vi "TEST_DSP.vi"() -> ()   [LabVIEW 2019]
panel:
  in  "error in (no error) 2":errorcluster
  out "Waveform Chart":cluster{"Data[0]":dbl, "Data[1]":dbl}(graph)
  in  "Voltage":dbl=5.0
  in  "Current":dbl=1.0
  in  "OCP Level":dbl=5.0 format="%#_13g"
  in  "OVP Level":dbl=10.0 format="%#_13g"
  out "Read Data":string="iDRC,DSP1500-30WE,702648,1.03.42\n"
  in  "port":refnum<visa-resource-name>="TCPIP0::192.168.0.14::HISLIP0::INSTR"
  in  "conntect":bool
  in  "disconntect":bool
  in  "READ":bool
  in  "STOP":bool
  in  "ON":bool
  in  "OFF":bool
  out "error out 3":errorcluster
  # "iDRC"
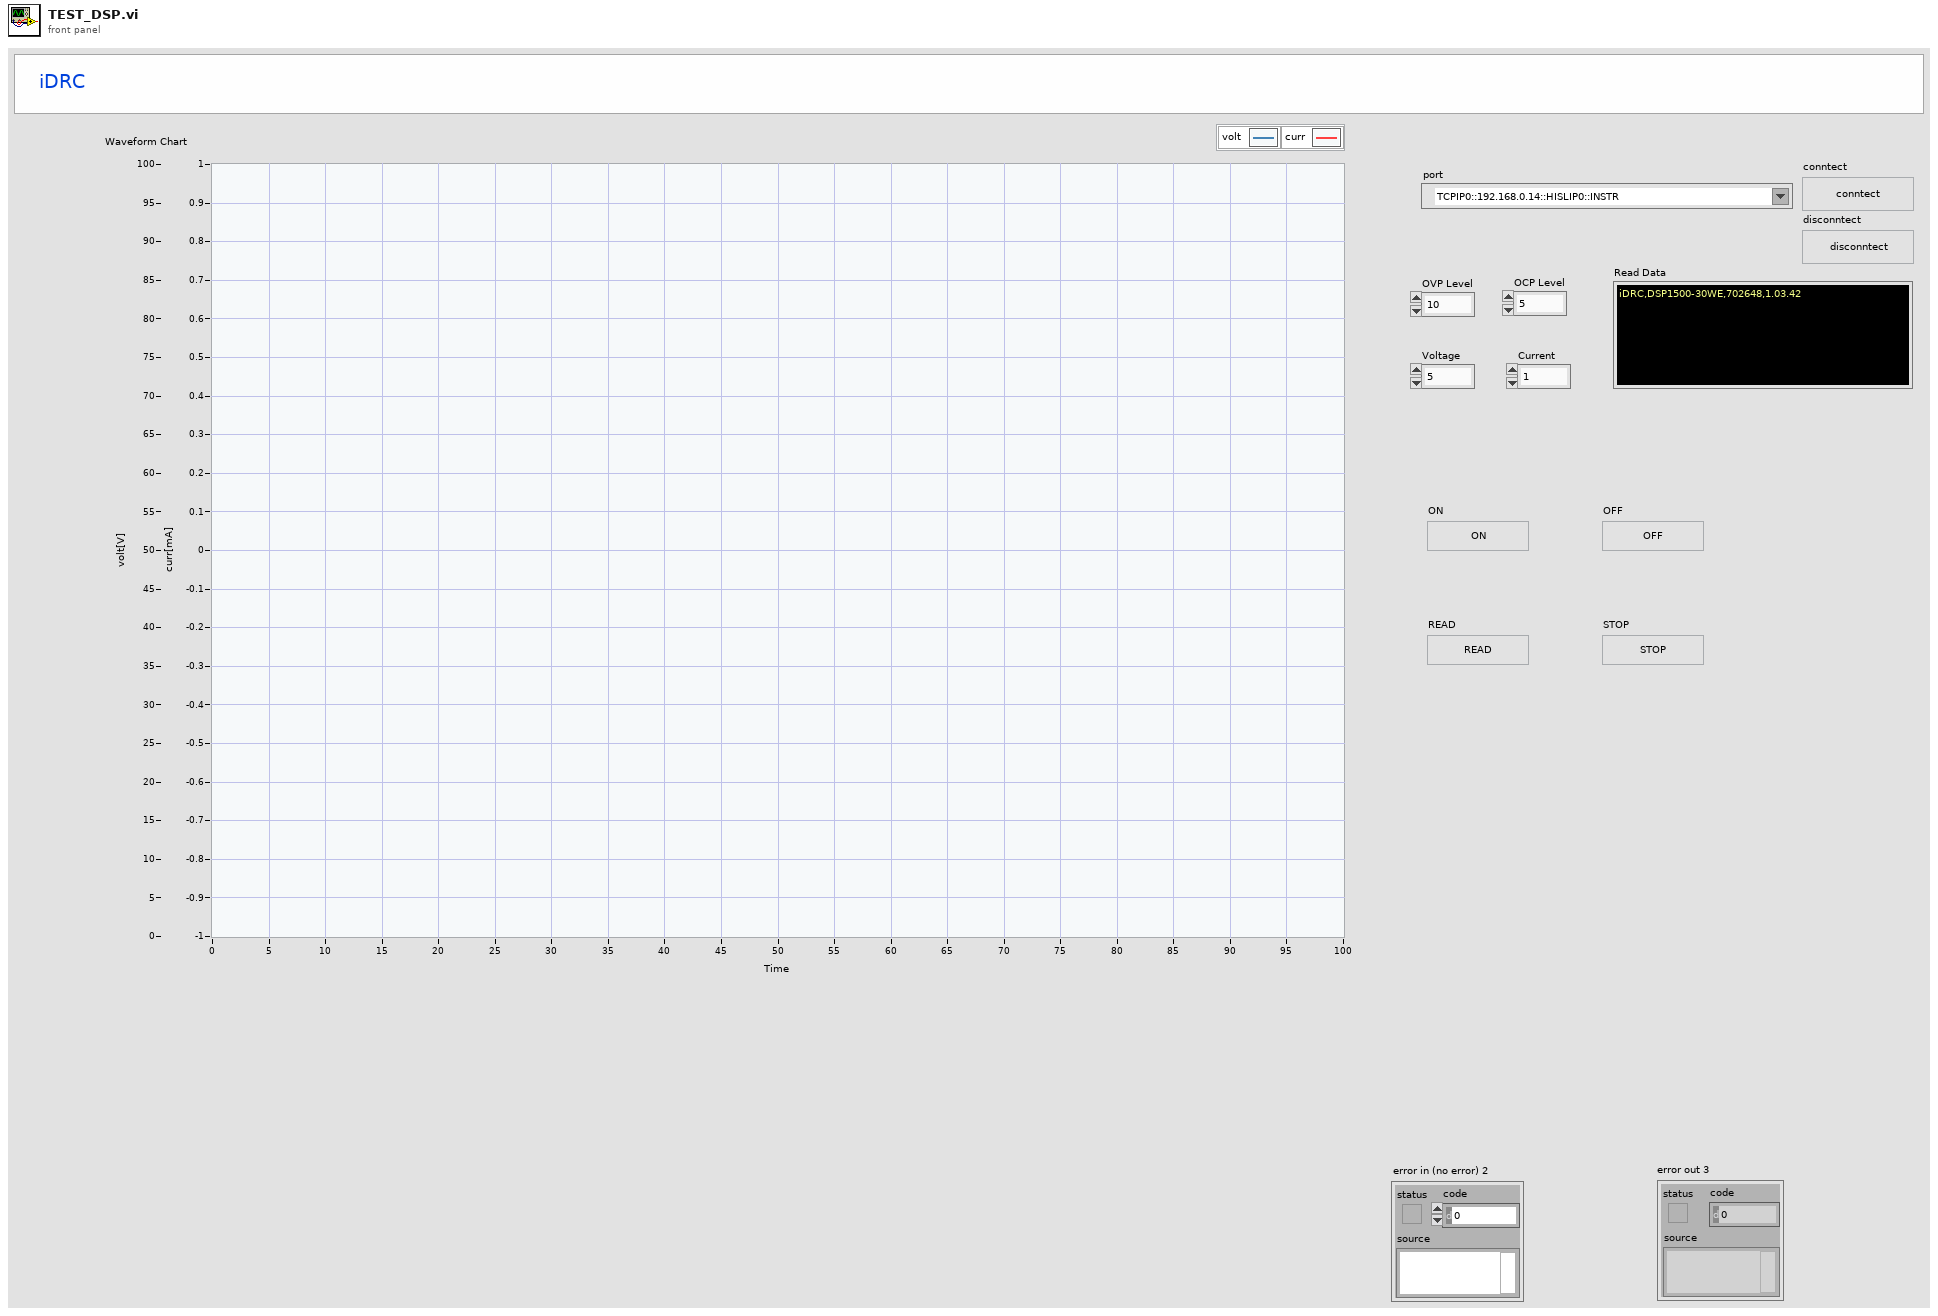
[diagram p1: front panel]
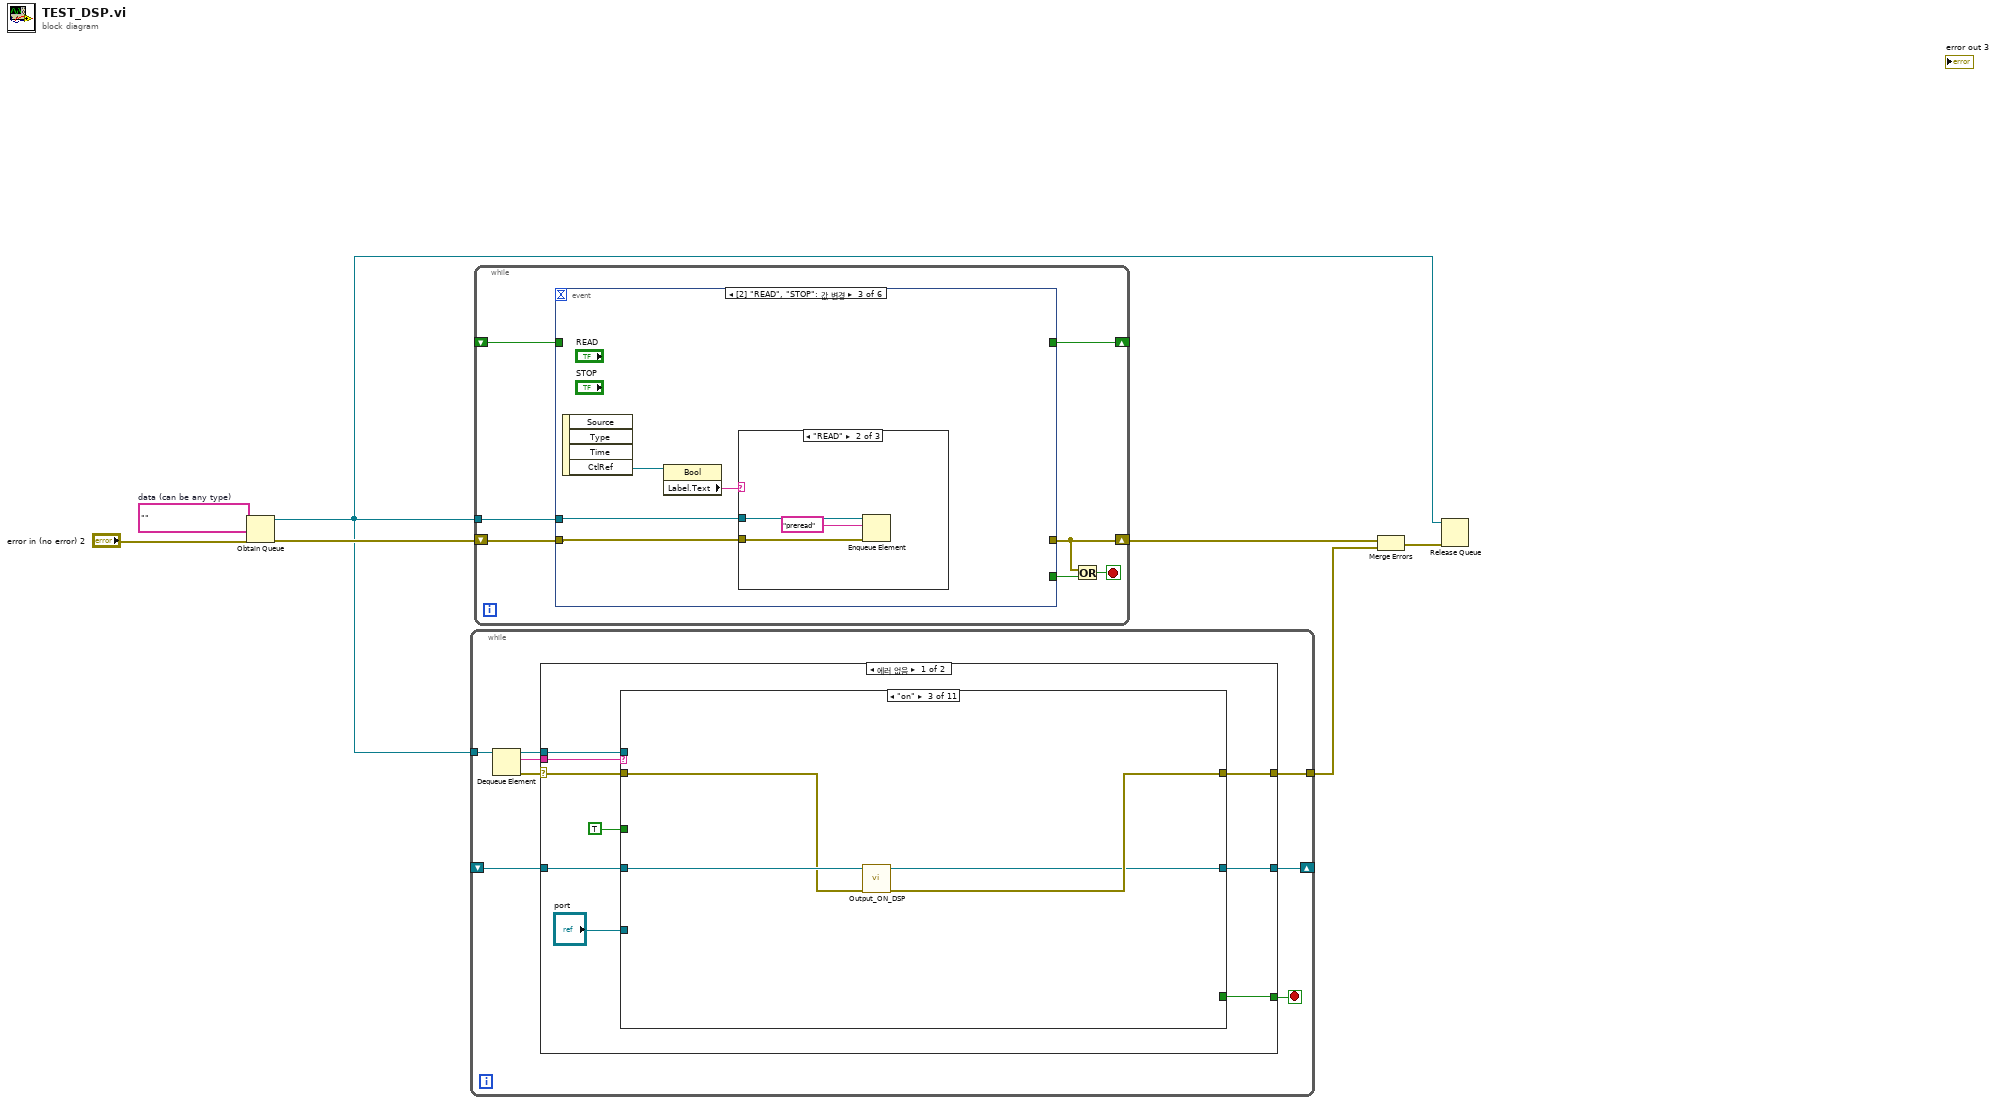
[diagram p0: block diagram]
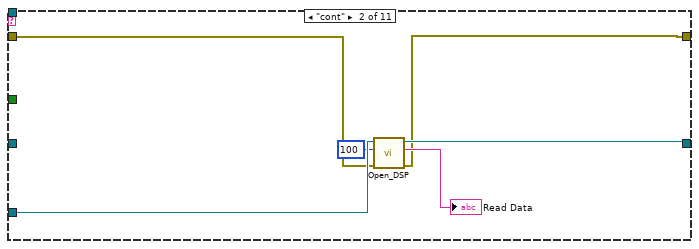
[diagram p3: hidden frame]
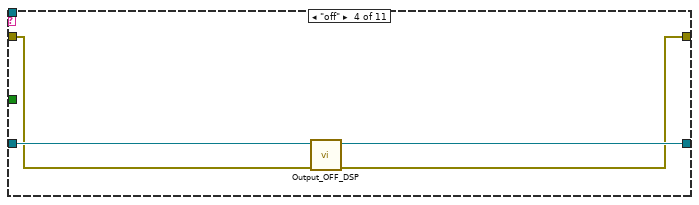
[diagram p4: hidden frame]
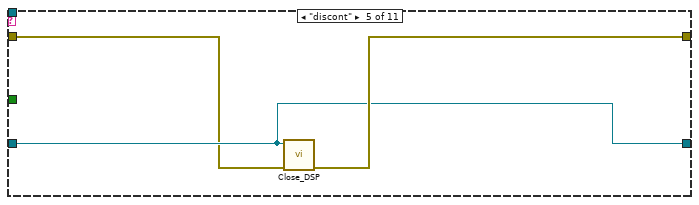
[diagram p5: hidden frame]
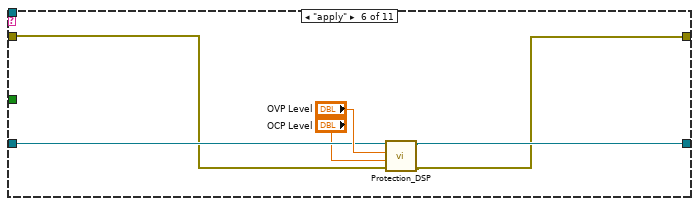
[diagram p6: hidden frame]
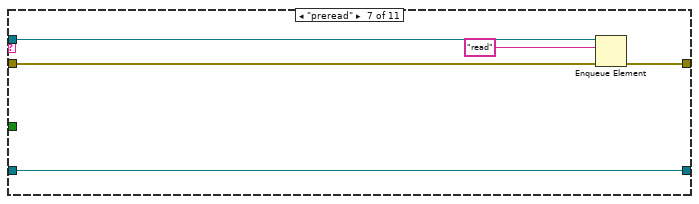
[diagram p7: hidden frame]
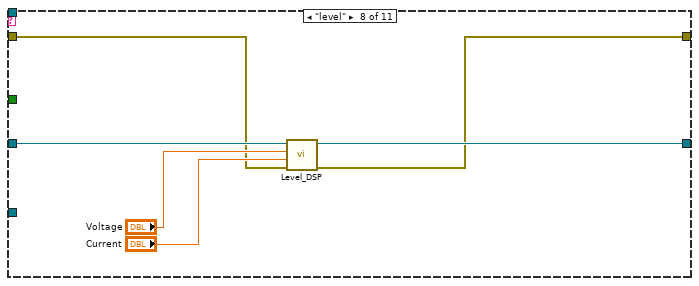
[diagram p8: hidden frame]
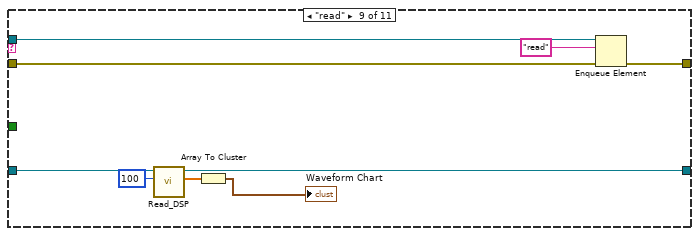
[diagram p9: hidden frame]
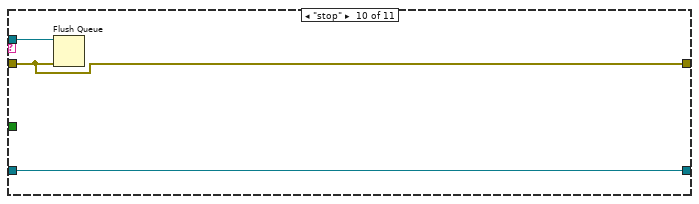
[diagram p10: hidden frame]
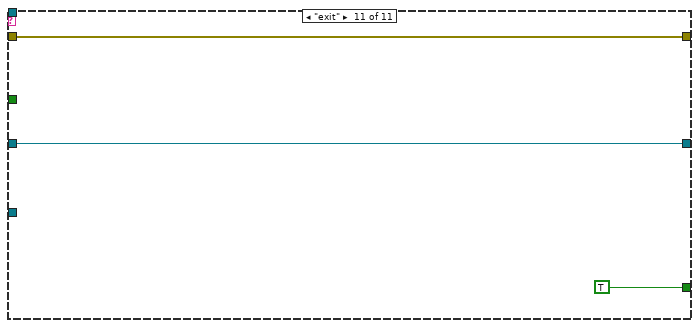
[diagram p11: hidden frame]
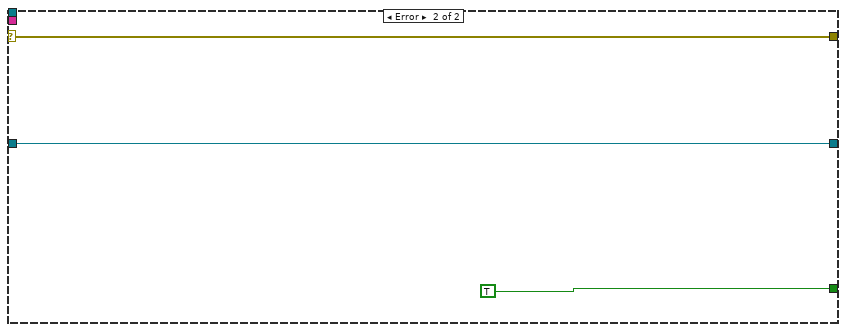
[diagram p12: hidden frame]
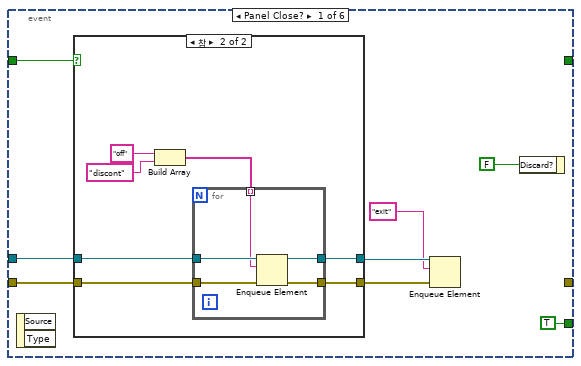
[diagram p13: hidden frame]
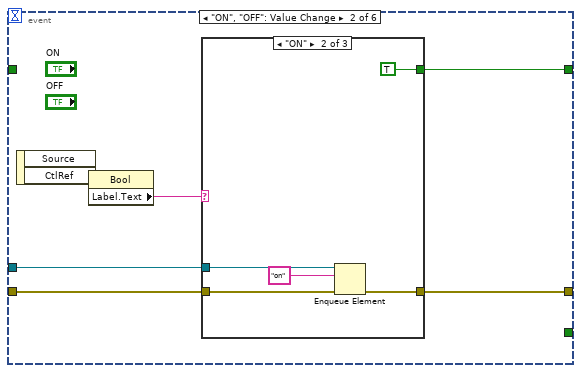
[diagram p15: hidden frame]
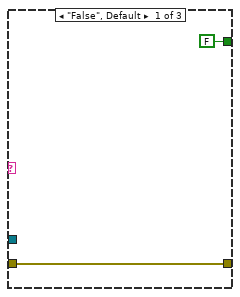
[diagram p16: hidden frame]
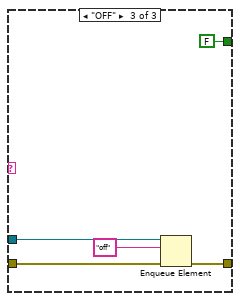
[diagram p17: hidden frame]
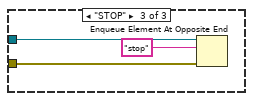
[diagram p19: hidden frame]
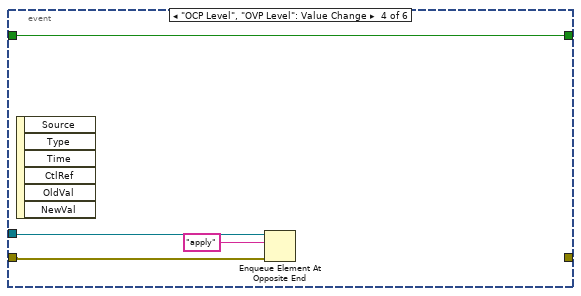
[diagram p20: hidden frame]
diagram:
  w6 = ""  # data (can be any type)
  n1 = Obtain Queue(element data type=w6, error in (no error)="error in (no error) 2") -> (queue out=w5:refnum<queue>, error out=w7:errorcluster)  [unwired: 3 in, 1 out]
  n2 = while {
    tunnel: w5 -> [w15]
    tunnel: [w10] -> w2
    shift-right: [w9] -> _
    shift-left: _ -> [w8]
    stop <- w12 stop-if-true
    n3 = Dequeue Element(queue=w15) -> (queue out=w11:refnum<queue>, element=w13:string, error out=w14:errorcluster)  [unwired: 2 in, 1 out]
    n4 = case shown="에러 없음" w14 {
      selector: w14 -> [w22 w77]
      tunnel: w13 -> [w24 _]
      tunnel: [w21 TRUE] -> w12
      tunnel: w11 -> [w23 _]
      tunnel: [w20 w77] -> w10
      tunnel: [w19 w76] -> w9
      tunnel: w8 -> [w18 w76]
      frame No Error {
        n5 = case shown="\"on\"" w24 {
          tunnel: w23 -> [_ _ _ _ _ _ w53 _ w69 w72 _]
          tunnel: w22 -> [w26 w29 w35 w38 w41 w46 w52 w56 w65 w71 w73]
          tunnel: [_ _ _ _ _ _ _ _ _ _ TRUE] -> w21
          tunnel: [w26 w28 w34 w37 w43 w45 w50 w55 w68 w71 w73] -> w20
          tunnel: [w25 w31 w33 w39 w42 w47 w51 w59 w66 w70 w74] -> w19
          tunnel: w18 -> [w25 _ w36 w40 w42 w48 w51 w60 w67 w70 w74]
          tunnel: "port" -> [_ w32 _ _ _ _ _ _ _ _ _]
          tunnel: TRUE -> [_ _ _ _ _ _ _ _ _ _ _]
          frame "False", Default {
          }
          frame "cont" {
            n6 = call "Open_DSP.vi"("error in"=w29, "Byte count"=u32 100, "VISA"=w32) -> ("error out"=w28:errorcluster, "read buffer"=→"Read Data":string, "VISA out"=w31:refnum<visa-resource-name>)  [unwired: 6 in]
          }
          frame "on" {
            n7 = call "Output_ON_DSP.vi"("error in"=w35, "VISA"=w36) -> ("error out"=w34:errorcluster, "VISA  Out"=w33:refnum<visa-resource-name>)  [unwired: 8 in]
          }
          frame "off" {
            n8 = call "Output_OFF_DSP.vi"("error in (no error)"=w38, "VISA resource name"=w40) -> ("error out"=w37:errorcluster, "VISA resource name Out"=w39:refnum<visa-resource-name>)  [unwired: 8 in]
          }
          frame "discont" {
            n9 = call "Close_DSP.vi"("error in (no error)"=w41, "VISA resource name"=w42) -> ("error out"=w43:errorcluster)  [unwired: 9 in]
          }
          frame "apply" {
            n10 = call "Protection_DSP.vi"("error in (no error)"=w46, "OCP Level"="OCP Level", "OVP Level"="OVP Level", "VISA resource name"=w48) -> ("error out"=w45:errorcluster, "VISA resource name Out"=w47:refnum<visa-resource-name>)  [unwired: 6 in]
          }
          frame "preread" {
            n11 = Enqueue Element(queue=w53, element="read", error in (no error)=w52) -> (error out=w50:errorcluster)  [unwired: 1 in, 2 out]
          }
          frame "level" {
            n12 = call "Level_DSP.vi"("error in (no error)"=w56, "Curr"="Current", "Volt"="Voltage", "VISA resource name"=w60) -> ("error out"=w55:errorcluster, "VISA resource name Out"=w59:refnum<visa-resource-name>)  [unwired: 6 in]
          }
          frame "read" {
            n13 = call "Read_DSP.vi"("Byte count"=u32 100, "port"=w67) -> ("Data"=w62:dbl[], "port Out"=w66:refnum<visa-resource-name>)  [unwired: 7 in, 1 out]
            n14 = Array To Cluster(array=w62) -> (cluster=→"Waveform Chart":cluster{"Data[0]":dbl, "Data[1]":dbl})
            n15 = Enqueue Element(queue=w69, element="read", error in (no error)=w65) -> (error out=w68:errorcluster)  [unwired: 1 in, 2 out]
          }
          frame "stop" {
            n16 = Flush Queue(queue=w72, error in (no error)=w71) -> ()  [unwired: 3 out]
          }
          frame "exit" {
          }
        }
      }
      frame Error {
      }
    }
  }
  n17 = while {
    shift-right: [w81] -> w3
    shift-left: w7 -> [w84]
    tunnel: w5 -> [w85]
    shift-right: [w80] -> _
    shift-left: _ -> [w79]
    stop <- w82 stop-if-true
    n18 = event shown="[2] \"READ\", \"STOP\": 값 변경" {
      selector: _ -> [_ _ _ _ _ _]
      dyn-events: _ -> [_ _ _ _ _ _]
      timeout: _ -> [_ _ _ _ _ _]
      tunnel: w85 -> [w90 w113 w129 w138 w142 w149]
      tunnel: w84 -> [w89 w112 w128 w137 w141 w148]
      tunnel: [_ w111 _ _ _ w147] -> w81
      tunnel: [TRUE ("stop") _ _ _ _ _] -> w83
      tunnel: [_ w108 _ w136 w140 w144] -> w80
      tunnel: w79 -> [w91 _ _ w136 w140 _]
      event Panel Close? {
        n19 = event-data() -> ()  [unwired: 1 in, 2 out]
        n20 = case shown="참" w91 {
          tunnel: w90 -> [w95 w100]
          tunnel: w89 -> [w94 w99]
          tunnel: [w95 w97] -> w88
          tunnel: [w94 w96] -> w87
          frame False {
          }
          frame True {
            n21 = Build Array("off" ("element"), "discont" ("element")) -> (w98:string[])
            n22 = for {
              tunnel: w100 -> [w107]
              tunnel: w99 -> [w106]
              tunnel: w98 -> [w105] mode=indexing
              tunnel: [w104] -> w97
              tunnel: [w103] -> w96
              n23 = Enqueue Element(queue=w107, element=w105, error in (no error)=w106) -> (queue out=w104:refnum<queue>, error out=w103:errorcluster)  [unwired: 1 in, 1 out]
            }
          }
        }
        n24 = Enqueue Element(queue=w88, element="exit", error in (no error)=w87) -> ()  [unwired: 1 in, 3 out]
        n25 = event-data("Discard?"=FALSE) -> ()  [unwired: 1 in, 1 out]
      }
      event "ON", "OFF": Value Change {
        n26 = event-data() -> ("CtlRef"=w110:refnum<vi>)  [unwired: 1 in, 1 out]
        n27 = property class="Bool"(reference=w110) -> ("Label.Text"=w109:string)  [unwired: 1 in, 2 out]
        n28 = case shown="\"ON\"" w109 {
          tunnel: w113 -> [_ w119 w124]
          tunnel: w112 -> [w115 w118 w123]
          tunnel: [w115 w117 w122] -> w111
          tunnel: [FALSE TRUE FALSE] -> w108
          frame "False", Default {
          }
          frame "ON" {
            n29 = Enqueue Element(queue=w119, element="on", error in (no error)=w118) -> (error out=w117:errorcluster)  [unwired: 1 in, 2 out]
          }
          frame "OFF" {
            n30 = Enqueue Element(queue=w124, element="off", error in (no error)=w123) -> (error out=w122:errorcluster)  [unwired: 1 in, 2 out]
          }
        }
      }
      event "READ", "STOP": Value Change {
        n31 = event-data() -> ("CtlRef"=w127:refnum<vi>)  [unwired: 1 in, 3 out]
        n32 = property class="Bool"(reference=w127) -> ("Label.Text"=w126:string)  [unwired: 1 in, 2 out]
        n33 = case shown="\"READ\"" w126 {
          tunnel: w129 -> [_ w131 w134]
          tunnel: w128 -> [_ w130 w133]
          frame "False", Default {
          }
          frame "READ" {
            n34 = Enqueue Element(queue=w131, element="preread", error in (no error)=w130) -> ()  [unwired: 1 in, 3 out]
          }
          frame "STOP" {
            n35 = Enqueue Element At Opposite End(queue=w134, element="stop", error in (no error)=w133) -> ()  [unwired: 1 in, 3 out]
          }
        }
      }
      event "OCP Level", "OVP Level": Value Change {
        n36 = event-data() -> ()  [unwired: 1 in, 6 out]
        n37 = Enqueue Element At Opposite End(queue=w138, element="apply", error in (no error)=w137) -> ()  [unwired: 1 in, 3 out]
      }
      event "Voltage", "Current": Value Change {
        n38 = event-data() -> ()  [unwired: 1 in, 6 out]
        n39 = Enqueue Element At Opposite End(queue=w142, element="level", error in (no error)=w141) -> ()  [unwired: 1 in, 3 out]
      }
      event "conntect", "disconntect": Value Change {
        n40 = event-data() -> ("CtlRef"=w146:refnum<vi>)  [unwired: 1 in, 1 out]
        n41 = property class="Bool"(reference=w146) -> ("Label.Text"=w145:string)  [unwired: 1 in, 2 out]
        n42 = case shown="\"disconntect\"" w145 {
          tunnel: w149 -> [_ w156 w161]
          tunnel: w148 -> [w151 w155 w160]
          tunnel: [w151 w154 w159] -> w147
          tunnel: [FALSE TRUE FALSE] -> w144
          frame "False", Default {
          }
          frame "conntect" {
            n43 = Enqueue Element(queue=w156, element="cont", error in (no error)=w155) -> (error out=w154:errorcluster)  [unwired: 1 in, 2 out]
          }
          frame "disconntect" {
            n44 = Enqueue Element(queue=w161, element="discont", error in (no error)=w160) -> (error out=w159:errorcluster)  [unwired: 1 in, 2 out]
          }
        }
      }
    }
    n45 = Or(x=w81, y=w83) -> (x .or. y?=w82:bool)
  }
  n46 = Merge Errors(w3, w2) -> (w1:errorcluster)
  n47 = Release Queue(queue=w5, error in (no error)=w1) -> ()  [unwired: 1 in, 3 out]
